vi "Camera Manager Get Camera Param.vi"(8 "error in (no error)":errorcluster, 9 "Value":string, 10 "NodeName":string, 11 "cameraId":i32) -> (0 "error out":errorcluster, 1 "Value out":string, 2 "NodeName out":string)   [LabVIEW 2017, in "PlayNitrideCameraComponet1010_4.lvlib"]
doc: "__declspec(dllexport) void CameraManager_GetCameraParam(int cameraId, char* NodeName, char* Value);"
uses:
  <userlib>/PlayNitrideCameraComponet1010_4/PlayNitrideCameraComponet1010_4.lvlib
  <userlib>/PlayNitrideCameraComponet1010_4/PlayNitrideCameraComponet.dll
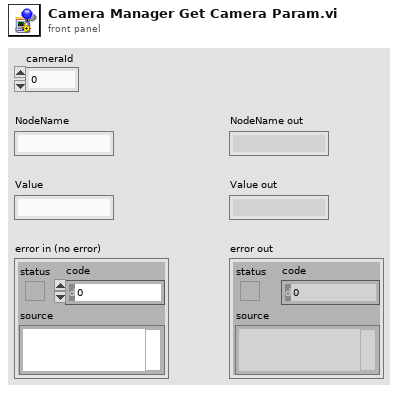
[diagram p1: front panel]
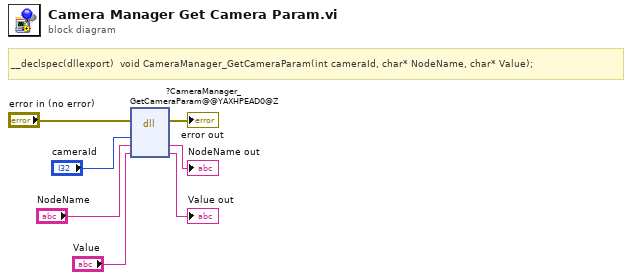
[diagram p0: block diagram]
diagram:
  # "__declspec(dllexport)  void CameraManager_GetCameraParam(int cameraId, char* NodeName, char* Value);"
  n1 = dll-call lib="C:/Program Files/National Instruments/LabVIEW 2017/user.lib/PlayNitrideCameraComponet1010_4/PlayNitrideCameraComponet.*" fn="?CameraManager_GetCameraParam@@YAXHPEAD0@Z"(error in="error in (no error)", "cameraId"="cameraId", "NodeName"="NodeName", "Value"="Value") -> (error out=→"error out":errorcluster, "NodeName"=→"NodeName out":string, "Value"=→"Value out":string)  [unwired: 4 in, 1 out]
